vi "crio_FPGA_Antagonist_Force.vi"() -> ()   [LabVIEW 2019]
uses:
  <vilib>/rvi/Analysis/control/PID/Typedef/niFpgaPID_ManualControl.ctl
  <vilib>/rvi/Analysis/control/PID/Typedef/niFpgaPID_PIGains.ctl
  <vilib>/LabVIEW Targets/FPGA/cRIO/shared/nicrio_ModuleControls/nicrio_cRIO-9237_ExcitationVoltageRing.ctl
  <vilib>/LabVIEW Targets/FPGA/cRIO/shared/nicrio_ModuleControls/nicrio_cRIO-9237_DataRatesRing.ctl
  <vilib>/rvi/Analysis/control/PID/Typedef/niFpgaPID_OutputRange.ctl
  <vilib>/rvi/Emulation/niFpgaSctlEmulationGetInTimedLoop.vi
  <vilib>/rvi/Emulation/niFpgaProcessEmulError.vi
  <vilib>/rvi/eio/common/nirviEmuTemplateMethod_errors.vi
  <vilib>/rvi/eio/common/nirviEmuTemplatePropertySet_errors.vi
  <vilib>/rvi/Emulation/niFpgaGetClockAttributes.vi
  <vilib>/rvi/Emulation/niFpgaEmulationReportErrorSimple.vi
  <vilib>/rvi/Emulation/niFpgaCriticalErrorInLSC.vi
  <vilib>/rvi/Analysis/control/PID/SubVIs/niFpgaPID_PIWrapper.vi
  <vilib>/eio/EIOMethodNode/EIOMethodNode.xnode
  <vilib>/eio/EIOPropertyNode/EIOPropertyNode.xnode
  <vilib>/eio/EIONode/EIONode.xnode
  <vilib>/rvi/FXPMathLib/FxpInterpret/XNode/nifxpmath_Interpret.xnode
  <vilib>/rvi/FXPMathLib/FxpMul/XNode/nifxpmath_Multiplier.xnode
  <vilib>/rvi/FXPMathLib/FxpAdd/XNode/nifxpmath_Add.xnode
  <vilib>/rvi/eio/common/nirviEmuTemplatePropertyGet_errors.vi
  <vilib>/rvi/eio/common/nirviEmuTemplatePropertyGet_noerrors.vi
  <vilib>/rvi/eio/common/nirviEmuTemplatePropertySet_noerrors.vi
  <vilib>/rvi/FXPMathLib/sim/FxpSim.dll
panel:
  in  "sweep frequency (periods/tick)":fxp<+,32,0>=1.25030055642128e-06
  out "sine out":i16
  out "sin_fxp":fxp<+/-,16,1>
  out "cosine out":i16
  in  "Lock_loop_rate":u32 caption="Count(uSec)"
  in  "sin_gain":fxp<+,32,10>
  in  "sin_offset":fxp<+/-,32,10>=0.5
  out "VCA Force Setpoint":sgl
  out "scaled load cell reading":fxp<+/-,24,24>
  out "error out":errorcluster {"code" format="%.0x"}
  in  "Finite?":bool=TRUE
  in  "Samples per Channel":u32=1000
  out "Mod1/AI0":fxp<+/-,24,-4>
  in  "Loop Rate (uSec)":u32
  in  "Shunt Cal Enable":bool
  in  "Data Rate":T1=1 items=["50.000 kS/s (NI 9237)"=1, "25.000 kS/s (NI 9237)"=2, "16.667 kS/s (NI 9237)"=3, "12.500 kS/s (NI 9237)"=4, "10.000 kS/s (NI 9237)"=5, "8.333 kS/s (NI 9237)"=6, "7.143 kS/s (NI 9237)"=7, "6.250 kS/s (NI 9237)"=8, "5.556 kS/s (NI 9237)"=9, "5.000 kS/s (NI 9237)"=10, "4.545 kS/s (NI 9237)"=11, "4.167 kS/s (NI 9237)"=12, "3.846 kS/s (NI 9237)"=13, "3.571 kS/s (NI 9237)"=14, "3.333 kS/s (NI 9237)"=15, "3.125 kS/s (NI 9237)"=16, "2.941 kS/s (NI 9237)"=17, "2.778 kS/s (NI 9237)"=18, "2.632 kS/s (NI 9237)"=19, "2.500 kS/s (NI 9237)"=20, "2.381 kS/s (NI 9237)"=21, "2.273 kS/s (NI 9237)"=22, "2.174 kS/s (NI 9237)"=23, "2.083 kS/s (NI 9237)"=24, "2.000 kS/s (NI 9237)"=25, "1.923 kS/s (NI 9237)"=26, "1.852 kS/s (NI 9237)"=27, "1.786 kS/s (NI 9237)"=28, "1.724 kS/s (NI 9237)"=29, "1.667 kS/s (NI 9237)"=30, "1.613 kS/s (NI 9237)"=31]
  in  "Excitation Voltage":T2 items=["2.5 Volts", "3.3 Volts", "5.0 Volts", "10.0 Volts", "External Excitation"]
  in  "Half-Bridge Enable":bool
  in  "LAC Lock":bool
  in  "VCA Gains":T3 {"proportional gain" step=0.125}
  in  "LAC DC PWM Period (us)":i16=50
  in  "Debug: ConnectorA/DIO15":bool
  in  "Debug: ConnectorA/DIO14":bool
  in  "Encoder Debug":bool
  in  "Loop Timer DAQ":u32=1 caption="LAC Loop Time(uSec)"
  in  "Position Reset":bool
  out "LAC Position (Counts)":i32
  out "LAC B":bool
  out "LAC A":bool
  out "LAC B'":bool
  out "LAC A'":bool
  in  "LAC Velocity Interval (uSec)":u32=1000
  out "LAC Acceleration (Counts/Interval)":i32
  out "LAC Velocity (Counts/Interval)":i32
  out "LAC Controller PWM Output":sgl
  in  "LAC Manual Control":T4 {"manual input (0)" scale=-1.0..1.0}
  in  "LAC Setpoint":i32
  in  "LAC Gains":T3={"proportional gain"=0.01, "integral gain"=6e-09} {"proportional gain" step=0.125}
  in  "rail Initial Position":i16=1
  out "rail Platform Position":i16
  in  "Stepper Direction":bool
  in  "Stepper Enable":bool
  in  "Position Control: Desired Positoin":i16=100
  in  "Manual Operation":bool
  out "Controller Enable":bool
  out "Controller Direction":bool
  in  "mSec to initialize a small push away from limit switch":u32=1 caption="mSec when hit limit"
  in  "mSec when hit limit":u32=100 caption="rail mSec to pause when hit limit"
  in  "Rail soft limit":i16=10000
  out "Limit Switch":bool
  in  "Half Peirod (pulse 40MHz)":u32=10000 caption="rail Count(Tick) [Interval between step]"
  out "VCA ControllerPWM Output":sgl
  in  "VCA Manual Control":T4 {"manual input (0)" scale=-1.0..1.0}
  in  "DC PWM Period (microsec)":i16=50
  in  "stop":bool=TRUE
  # "Period Default 500(us) 2kHz"
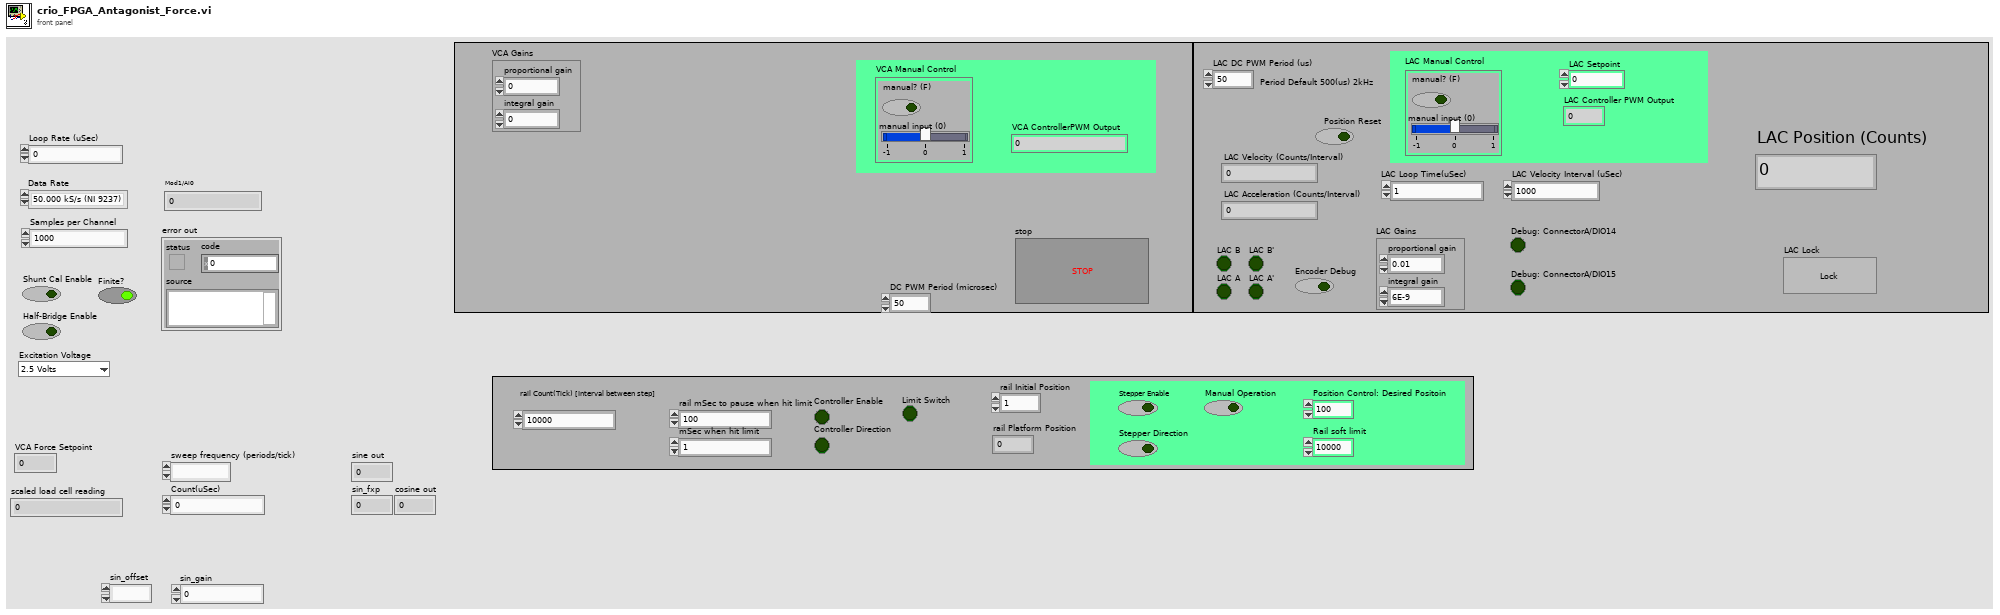
[diagram p1: front panel]
types:
  T1 = typedef "nicrio_cRIO-9237_DataRatesRing.ctl" = u8
  T2 = typedef "nicrio_cRIO-9237_ExcitationVoltageRing.ctl" = u8
  T3 = typedef "niFpgaPID_PIGains.ctl" = cluster{"proportional gain":sgl, "integral gain":sgl}
  T4 = typedef "niFpgaPID_ManualControl.ctl" = cluster{"manual? (F)":bool, "manual input (0)":sgl}
  T5 = typedef "niFpgaPID_OutputRange.ctl" = cluster{"output high (Inf)":sgl, "output low (-Inf)":sgl}
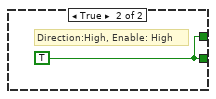
[diagram p6: hidden frame]
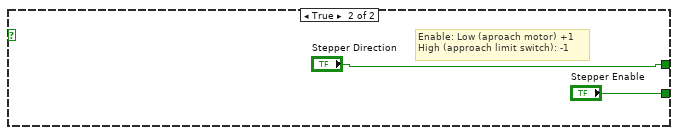
[diagram p7: hidden frame]
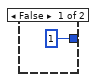
[diagram p9: hidden frame]
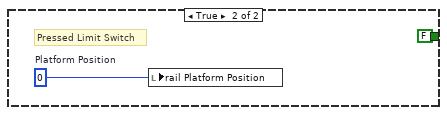
[diagram p11: hidden frame]
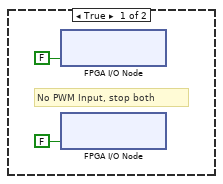
[diagram p13: hidden frame]
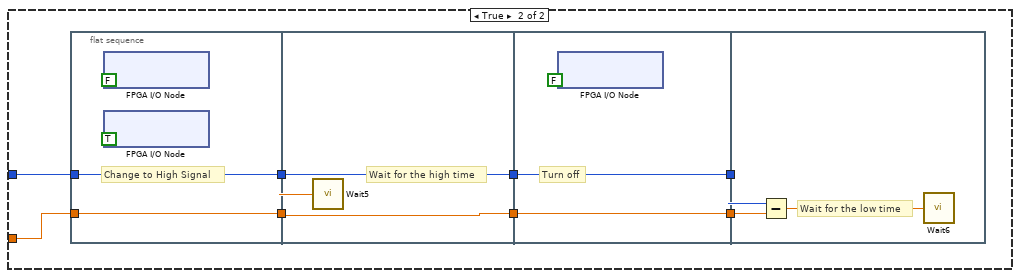
[diagram p14: hidden frame]
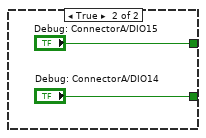
[diagram p17: hidden frame]
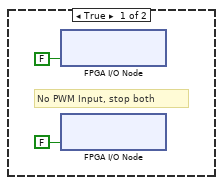
[diagram p18: hidden frame]
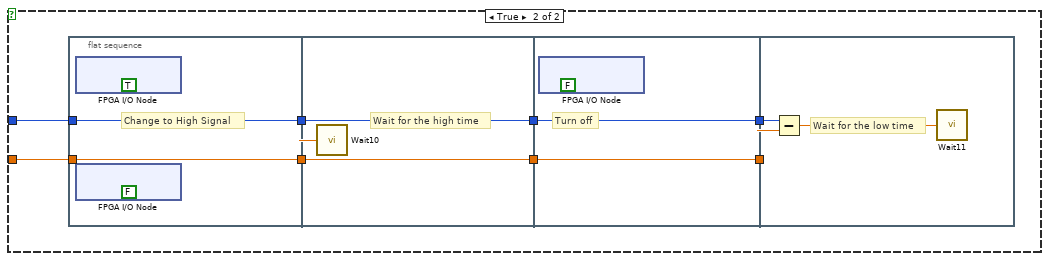
[diagram p19: hidden frame]
diagram:
  n1 = flat-sequence {
    tunnel: [w6] -> w2
    tunnel: [w5] -> w1
    tunnel: w2 -> [w30]
    tunnel: w1 -> [w29]
    frame #0 {
      n2 = disable-structure shown="Enabled" {
        disable-tunnel: [w17 _] -> w6
        disable-tunnel: ["Data Rate" _] -> w5
        frame Enabled {
          # "red to 2\ngreen to 3\nblack to 21\nwhite to 22"
          # "Start the Aquisition"
          # "For Quarter and Half Bridge strain gauges enable the half bridge \nto complete the full bridge."
          # "Set the modules data rate, acquisition rate, and excitation voltage."
          n3 = xnode "FPGA I/O Property Node"("error in"=errorcluster {"status"=FALSE, "code"=0, "source"=""}, "Data Rate"="Data Rate", "Excitation Voltage"="Excitation Voltage") -> ("error out"=w27:errorcluster)  [unwired: 1 in, 1 out]
          n4 = xnode "FPGA I/O Property Node"("error in"=w27, "Half-Bridge Enable"="Half-Bridge Enable") -> ("error out"=w23:errorcluster)  [unwired: 1 in, 1 out]
          n5 = xnode "FPGA I/O Property Node"("error in"=w27, "Half-Bridge Enable"="Half-Bridge Enable") -> ("error out"=w24:errorcluster)  [unwired: 1 in, 1 out]
          n6 = xnode "FPGA I/O Property Node"("error in"=w27, "Half-Bridge Enable"="Half-Bridge Enable") -> ("error out"=w25:errorcluster)  [unwired: 1 in, 1 out]
          n7 = xnode "FPGA I/O Property Node"("error in"=w27, "Half-Bridge Enable"="Half-Bridge Enable") -> ("error out"=w26:errorcluster)  [unwired: 1 in, 1 out]
          n8 = local write "Loop Rate (uSec)"(u32 100 ("Loop Rate (uSec)")) -> ()
          n9 = Merge Errors(w23, w24, w25, w26) -> (w28:errorcluster)
          n10 = xnode "FPGA I/O Node"("error in"=w28, "Mod6/Start"=TRUE ("Mod1/Stop")) -> ("error out"=w17:errorcluster)  [unwired: 1 in, 1 out]
        }
        frame Disabled {
        }
      }
      n11 = local write "scaled load cell reading"(0 ("LAC Position (Counts)")) -> ()
      n12 = local write "VCA Force Setpoint"(0 ("LAC Position (Counts)")) -> ()
      n13 = local write "stop"(FALSE ("stop")) -> ()
      n14 = xnode "FPGA I/O Method Node"("DIO 7:4"=enum8{"No Change", "Input", "Output"}."Input", "DIO 3:0"=enum8{"No Change", "Input", "Output"}."Output") -> ()  [unwired: 1 in, 1 out]
      n15 = local write "LAC Controller PWM Output"(u32 0 ("Servo wait time")) -> ()
      n16 = local write "LAC Position (Counts)"(0 ("LAC Position (Counts)")) -> ()
      n17 = local write "Encoder Debug"(FALSE ("LAC Lock")) -> ()
      n18 = local write "LAC Lock"(FALSE ("LAC Lock")) -> ()
      n19 = xnode "FPGA I/O Method Node"("Enable"=u8 0) -> ()  [unwired: 1 in, 1 out]
      "rail Platform Position" <- "rail Initial Position"
    }
    frame #1 {
      n20 = disable-structure shown="Enabled" {
        disable-tunnel: w30 -> [w32 _]
        disable-tunnel: w29 -> [w31 _]
        frame Enabled {
          n21 = while {
            stop <- w36 stop-if-true
            # "Shift by 20 bits"
            # "output"
            # "PWM"
            # "current offset"
            # "sine wave amplitude"
            # "Lock in"
            n22 = local read "Mod1/AI0"() -> (w35:fxp<+/-,24,-4>)
            n23 = call "Loop Timer2"("Count(uSec)"="Lock_loop_rate") -> ()  [unwired: 1 out]
            n24 = xnode "Reinterpret Number"("x"=w35) -> ("y"=→"scaled load cell reading":fxp<+/-,24,16>)
            n25 = call "Sine Wave Generator"("frequency (periods/tick)"="sweep frequency (periods/tick)") -> ("sine out"=w45:i16, "cosine out"=→"cosine out":i16)  [unwired: 13 in]
            "sine out" <- w45
            n26 = xnode "Reinterpret Number"("x"=w45) -> ("y"=w42:fxp<+/-,16,1>)
            "sin_fxp" <- w42
            n27 = xnode ("High Throughput Multiply")("x"=w42, "y"="sin_gain") -> ("x*y"=w40:fxp<+/-,48,11>)
            n28 = xnode ("High Throughput Add")("x"=w40, "y"="sin_offset") -> ("x+y"=w38:fxp<+/-,49,12>)
            n29 = To Single Precision Float(number=w38) -> (single precision float=→"VCA Force Setpoint":sgl)
            n30 = local read "stop"() -> (w36:bool)
          }
          n31 = flat-sequence {
            tunnel: [w49] -> w33
            tunnel: w32 -> [w48]
            tunnel: w31 -> [w47]
            tunnel: w33 -> [w118]
            frame #0 {
              # "Stop on any error or if the stop Boolean is true"
              n32 = while {
                tunnel: w48 -> [w60]
                tunnel: [w57] -> w49
                tunnel: w47 -> [w55]
                stop <- w58 stop-if-true
                n33 = flat-sequence {
                  tunnel: [w63] -> w56
                  tunnel: [w62] -> w53
                  tunnel: ["Shunt Cal Enable"] -> w52
                  tunnel: w55 -> [w62]
                  tunnel: w60 -> [w64]
                  tunnel: [w81] -> w59
                  tunnel: w56 -> [w82]
                  tunnel: [w80] -> w54
                  tunnel: w53 -> [w80]
                  tunnel: w52 -> [w79]
                  tunnel: [w79] -> w51
                  tunnel: [w101] -> w57
                  tunnel: w59 -> [w102]
                  tunnel: w54 -> [w99]
                  tunnel: w51 -> [w100]
                  frame #0 {
                    n34 = case shown="True" "Shunt Cal Enable" {
                      tunnel: w64 -> [w65 w75]
                      tunnel: [w65 w73] -> w63
                      tunnel: w62 -> [_ w70]
                      frame False {
                      }
                      frame True {
                        w68 = TRUE ("Shunt Cal Enable")
                        # "If Shunt Cal Enable is true stop the acquisition, switch on the shunt resistors, set the data rate and begin the acquisition."
                        n35 = xnode "FPGA I/O Node"("error in"=w75, "Mod6/Stop"=TRUE ("Mod1/Stop")) -> ("error out"=w74:errorcluster)  [unwired: 1 in, 1 out]
                        n36 = xnode "FPGA I/O Property Node"("error in"=w74, "Shunt Cal Enable"=w68) -> ("error out"=w78:errorcluster)  [unwired: 1 in, 1 out]
                        n37 = xnode "FPGA I/O Property Node"("error in"=w74, "Shunt Cal Enable"=w68) -> ("error out"=w66:errorcluster)  [unwired: 1 in, 1 out]
                        n38 = xnode "FPGA I/O Property Node"("error in"=w74, "Shunt Cal Enable"=w68) -> ("error out"=w77:errorcluster)  [unwired: 1 in, 1 out]
                        n39 = xnode "FPGA I/O Property Node"("error in"=w74, "Shunt Cal Enable"=w68) -> ("error out"=w76:errorcluster)  [unwired: 1 in, 1 out]
                        n40 = Merge Errors(w78, w66, w77, w76) -> (w71:errorcluster)
                        n41 = xnode "FPGA I/O Property Node"("error in"=w71, "Data Rate"=w70) -> ("error out"=w72:errorcluster)  [unwired: 1 in, 1 out]
                        n42 = xnode "FPGA I/O Node"("error in"=w72, "Mod6/Start"=TRUE ("Mod1/Start")) -> ("error out"=w73:errorcluster)  [unwired: 1 in, 1 out]
                      }
                    }
                  }
                  frame #1 {
                    n43 = while {
                      tunnel: w82 -> [w84]
                      tunnel: [w88] -> w81
                      i -> [w92]
                      stop <- w85 stop-if-true
                      # "When the Finite Boolean is true the code will acquire a discrete set of values in order to perform the offset null and/or shunt calibration otherwise the loop continuously acquires data."
                      n44 = Decrement(x="Samples per Channel") -> (x-1=w94:u32)
                      n45 = call "Loop Timer3"("Count(uSec)"="Loop Rate (uSec)") -> ()  [unwired: 1 out]
                      n46 = To Unsigned Long Integer(number=w92) -> (unsigned 32bit integer=w93:u32)
                      n47 = Equal?(x=w94, y=w93) -> (x = y?=w89:bool)
                      n48 = xnode "FPGA I/O Node"("error in"=w84) -> ("error out"=w88:errorcluster, "Mod6/AI0"=w98:fxp<+/-,24,-4>, "Mod6/AI1"=w97:fxp<+/-,24,-4>, "Mod6/AI2"=w95:fxp<+/-,24,-4>, "Mod6/AI3"=w96:fxp<+/-,24,-4>)  [unwired: 4 in, 4 out]
                      "Mod1/AI0" <- w98
                      n49 = And(x="Finite?", y=w89) -> (x .and. y?=w87:bool)
                      n50 = Build Array(w98, w97, w95, w96) -> ()  [unwired: 1 out]
                      n51 = local read "stop"() -> (w86:bool)
                      n52 = Compound Arithmetic op=OR(w88, w87, w86) -> (w85:bool)
                    }
                  }
                  frame #2 {
                    n53 = case shown="True" w100 {
                      tunnel: w102 -> [w103 w112]
                      tunnel: [w103 w110] -> w101
                      tunnel: w99 -> [_ w107]
                      frame False {
                      }
                      frame True {
                        w106 = FALSE ("Shunt Cal Enable")
                        # "If shunt calibration is set to true, data has been collected to perform the calibration. Next the acquisition is stopped, and then we switch off the shunt resistors, set the data rate, and start the acquisition."
                        n54 = xnode "FPGA I/O Node"("error in"=w112, "Mod6/Stop"=TRUE ("Mod1/Stop")) -> ("error out"=w111:errorcluster)  [unwired: 1 in, 1 out]
                        n55 = xnode "FPGA I/O Property Node"("error in"=w111, "Shunt Cal Enable"=w106) -> ("error out"=w116:errorcluster)  [unwired: 1 in, 1 out]
                        n56 = xnode "FPGA I/O Property Node"("error in"=w111, "Shunt Cal Enable"=w106) -> ("error out"=w115:errorcluster)  [unwired: 1 in, 1 out]
                        n57 = xnode "FPGA I/O Property Node"("error in"=w111, "Shunt Cal Enable"=w106) -> ("error out"=w114:errorcluster)  [unwired: 1 in, 1 out]
                        n58 = xnode "FPGA I/O Property Node"("error in"=w111, "Shunt Cal Enable"=w106) -> ("error out"=w113:errorcluster)  [unwired: 1 in, 1 out]
                        n59 = Merge Errors(w116, w115, w114, w113) -> (w108:errorcluster)
                        n60 = xnode "FPGA I/O Property Node"("error in"=w108, "Data Rate"=w107) -> ("error out"=w109:errorcluster)  [unwired: 1 in, 1 out]
                        n61 = xnode "FPGA I/O Node"("error in"=w109, "Mod6/Start"=TRUE ("Mod1/Start")) -> ("error out"=w110:errorcluster)  [unwired: 1 in, 1 out]
                      }
                    }
                  }
                }
                n62 = local read "stop"() -> (w50:bool)
                n63 = Or(x=w57, y=w50) -> (x .or. y?=w58:bool)
              }
            }
            frame #1 {
              # "Stop the acquisition and display any errors that occurred."
              n64 = xnode "FPGA I/O Node"("error in"=w118, "Mod6/Stop"=TRUE ("Mod1/Stop")) -> ("error out"=→"error out":errorcluster)  [unwired: 1 in, 1 out]
            }
          }
        }
        frame Disabled {
        }
      }
      n65 = disable-structure "LAC Position Control" shown="Enabled" {
        frame Enabled {
          n66 = while "Input Loop" {
            shift-right: [w254] -> _
            shift-left: _ -> [w257]
            shift-right: [w253] -> _
            shift-left: _ -> [w256]
            shift-right: [w249] -> _
            shift-left: _ -> [w255]
            shift-right: [w242] -> _
            shift-left: _ -> [w252]
            shift-right: [w243] -> _
            shift-left: _ -> [w251]
            shift-right: [w250] -> _
            shift-left: _ -> [w248]
            shift-right: [w247] -> _
            shift-left: _ -> [w246]
            shift-right: [w245] -> _
            shift-left: _ -> [w244]
            stop <- w241 stop-if-true
            # "B'"
            # ">>ChB>>"
            # ">>ChA>>"
            # "A'"
            # "A  -> Current Quadrature Encoder Channel A value\nA' -> Last value of Quadrature Encoder Channel A\nB  -> Current Quadrature Encoder Channel B value\nB' -> Last value of Quadrature Encoder Channel B"
            # "B'"
            # "B"
            # "A"
            n67 = case "Debug Input" shown="False" "Encoder Debug" {
              tunnel: [w275 "Debug: ConnectorA/DIO15"] -> w253
              tunnel: [w274 "Debug: ConnectorA/DIO14"] -> w254
              frame False {
                n68 = xnode "FPGA I/O Node"() -> ("Mod2/DIO2"=w275:bool, "Mod2/DIO3"=w274:bool)  [unwired: 2 in, 2 out]
              }
              frame True {
              }
            }
            "LAC B" <- w254
            "LAC A" <- w253
            n69 = call "Loop Timer"("Count(uSec)"="Loop Timer DAQ") -> ()  [unwired: 1 out]
            n70 = call "subvi_encoder_update.vi"("Position Reset"="Position Reset", "Tick'"=w255, "A"=w253, "B'"=w257, "A'"=w256, "B"=w254) -> ("Tick"=w249:i32)  [unwired: 5 in]
            "LAC Position (Counts)" <- w249
            n71 = disable-structure shown="Enabled" {
              disable-tunnel: w252 -> [w272 _]
              disable-tunnel: w251 -> [w271 _]
              disable-tunnel: [w270 _] -> w250
              disable-tunnel: w249 -> [w269 _]
              disable-tunnel: w248 -> [w268 _]
              disable-tunnel: [w267 _] -> w247
              disable-tunnel: w246 -> [w266 _]
              disable-tunnel: [w265 _] -> w245
              disable-tunnel: w244 -> [w264 _]
              disable-tunnel: [w262 _] -> w243
              disable-tunnel: [w261 _] -> w242
              frame Enabled {
                n72 = call "Time Count"() -> ("Tick Count(uSec)"=w263:u32)
                n73 = call "subvi_encoder_tick_to_pos.vi"("Velocity Interval (uSec)"="LAC Velocity Interval (uSec)", "Raw Tick"=w269, "Waited?'"=w266, "Tick Count(uSec)'"=w264, "p'"=w268, "Time Count"=w263, "a'"=w271, "v'"=w272) -> ("Waited?"=w267:bool, "Tick Count(uSec)"=w265:u32, "p"=w270:i32, "a"=w262:i32, "v"=w261:i32)  [unwired: 3 in]
                "LAC Acceleration (Counts/Interval)" <- w262
                "LAC Velocity (Counts/Interval)" <- w261
              }
              frame Disabled {
              }
            }
            n74 = local read "stop"() -> (w241:bool)
            "LAC B'" <- w257
            "LAC A'" <- w256
          }
          n75 = while {
            stop <- w240 stop-if-true
            n76 = local read "LAC Position (Counts)"() -> (w239:i32)
            n77 = call-poly <vilib>:"niFpgaPID_Wrapper.vi"("setpoint"="LAC Setpoint", "process variable"=w239, "manual control"="LAC Manual Control", "gains"="LAC Gains", "output range"=T5 {"output high (Inf)"=1.0, "output low (-Inf)"=-1.0}) -> ("output"=→"LAC Controller PWM Output":sgl)  [unwired: 8 in, 2 out]
            n78 = local read "stop"() -> (w240:bool)
          }
          n79 = while "PWM Output Loop" {
            stop <- w278 stop-if-true
            # "PWM input range:\n[-1,1]"
            # "DRV8256 Specs:\n\n0 0: Brake Low\n1 1: Brake High\nPWM 0\n0 PWM"
            # "controller output"
            n80 = local read "LAC Controller PWM Output"() -> (w279:sgl)
            n81 = Multiply(x="LAC DC PWM Period (us)", y=w279) -> (x*y=w281:sgl)
            n82 = Greater?(x=w279, y=i16 0) -> (0:w282:bool)
            n83 = case shown="False" w282 {
              tunnel: w281 -> [w286 w317]
              tunnel: "LAC DC PWM Period (us)" -> [w284 w316]
              frame False {
                n84 = Equal To 0?(x=w286) -> (x = 0?=w285:bool)
                n85 = case shown="False" w285 {
                  tunnel: w286 -> [_ w296]
                  tunnel: w284 -> [_ w289]
                  frame True {
                    # "No PWM Input, stop both"
                    n86 = xnode "FPGA I/O Node"("Mod1/DIO2"=FALSE) -> ()  [unwired: 1 in, 1 out]
                    n87 = xnode "FPGA I/O Node"("Mod1/DIO3"=FALSE) -> ()  [unwired: 1 in, 1 out]
                  }
                  frame False {
                    # "Negative duty cycle (change direction by outputting to other PIN)"
                    n88 = flat-sequence {
                      tunnel: w296 -> [w299]
                      tunnel: [w298] -> w295
                      tunnel: [w297] -> w290
                      tunnel: w289 -> [w297]
                      tunnel: w295 -> [w303]
                      tunnel: [w303] -> w294
                      tunnel: [w302] -> w291
                      tunnel: w290 -> [w302]
                      tunnel: w294 -> [w305]
                      tunnel: [w305] -> w293
                      tunnel: [w304] -> w292
                      tunnel: w291 -> [w304]
                      tunnel: w293 -> [w309]
                      tunnel: w292 -> [w308]
                      frame #0 {
                        # "Change to High Signal"
                        n89 = xnode "FPGA I/O Node"("Mod1/DIO3"=TRUE) -> ()  [unwired: 1 in, 1 out]
                        n90 = xnode "FPGA I/O Node"("Mod1/DIO2"=FALSE) -> ()  [unwired: 1 in, 1 out]
                        n91 = Negate(x=w299) -> (-x=w298:sgl)
                      }
                      frame #1 {
                        # "Wait for the High Time"
                        n92 = call "Wait"("Count(uSec)"=w303) -> ()  [unwired: 1 out]
                      }
                      frame #2 {
                        # "Change to Low Signal"
                        n93 = xnode "FPGA I/O Node"("Mod1/DIO2"=FALSE) -> ()  [unwired: 1 in, 1 out]
                      }
                      frame #3 {
                        # "Wait for the low time"
                        n94 = Subtract(x=w308, y=w309) -> (x-y=w307:sgl)
                        n95 = call "Wait2"("Count(uSec)"=w307) -> ()  [unwired: 1 out]
                      }
                    }
                  }
                }
              }
              frame True {
                n96 = flat-sequence {
                  tunnel: w317 -> [w318]
                  tunnel: w316 -> [w319]
                  tunnel: [w319] -> w313
                  tunnel: [w318] -> w312
                  tunnel: [w323] -> w314
                  tunnel: w313 -> [w323]
                  tunnel: w312 -> [w322]
                  tunnel: [w322] -> w311
                  tunnel: [w325] -> w315
                  tunnel: w314 -> [w325]
                  tunnel: w311 -> [w324]
                  tunnel: [w324] -> w310
                  tunnel: w315 -> [w329]
                  tunnel: w310 -> [w327]
                  frame #0 {
                    # "Change to High Signal"
                    n97 = xnode "FPGA I/O Node"("Mod1/DIO2"=TRUE) -> ()  [unwired: 1 in, 1 out]
                    n98 = xnode "FPGA I/O Node"("Mod1/DIO3"=FALSE ("ConnectorB/DIO9")) -> ()  [unwired: 1 in, 1 out]
                  }
                  frame #1 {
                    # "Wait for the high time"
                    n99 = call "Wait10"("Count(uSec)"=w322) -> ()  [unwired: 1 out]
                  }
                  frame #2 {
                    # "Turn off"
                    n100 = xnode "FPGA I/O Node"("Mod1/DIO2"=FALSE) -> ()  [unwired: 1 in, 1 out]
                  }
                  frame #3 {
                    # "Wait for the low time"
                    n101 = Subtract(x=w329, y=w327) -> (x-y=w328:sgl)
                    n102 = call "Wait11"("Count(uSec)"=w328) -> ()  [unwired: 1 out]
                  }
                }
              }
            }
            n103 = local read "stop"() -> (w278:bool)
          }
          n104 = while {
            stop <- w233 stop-if-true
            # "Lock the LAC controller with relay.\nRelay pin HIGH means connects to ground, meaning LAC powered OFF."
            n105 = xnode "FPGA I/O Node"("Mod8/DIO6"="LAC Lock") -> ()  [unwired: 1 in, 1 out]
            n106 = local read "stop"() -> (w233:bool)
          }
        }
        frame Disabled {
        }
      }
      n107 = disable-structure "VCA Control" shown="Enabled" {
        frame Enabled {
          n108 = while {
            stop <- w179 stop-if-true
            n109 = local read "scaled load cell reading"() -> (w174:fxp<+/-,24,24>)
            n110 = local read "VCA Force Setpoint"() -> (w173:sgl)
            n111 = call-poly <vilib>:"niFpgaPID_Wrapper.vi"("setpoint"=w173, "process variable"=w174, "manual control"="VCA Manual Control", "gains"="VCA Gains", "output range"=T5 {"output high (Inf)"=1.0, "output low (-Inf)"=-1.0}) -> ("output"=→"VCA ControllerPWM Output":sgl)  [unwired: 8 in, 2 out]
            n112 = local read "stop"() -> (w179:bool)
          }
          n113 = while "PWM Output Loop" {
            stop <- w180 stop-if-true
            # "PWM input range:\n[-1,1]"
            # "DRV8256 Specs:\n\n0 0: Brake Low\n1 1: Brake High\nPWM 0\n0 PWM"
            # "controller output"
            n114 = local read "VCA ControllerPWM Output"() -> (w181:sgl)
            n115 = Greater?(x=w181, y=i16 0) -> (0:w184:bool)
            n116 = Multiply(x="DC PWM Period (microsec)", y=w181) -> (x*y=w183:sgl)
            n117 = case shown="False" w184 {
              tunnel: w183 -> [w188 w219]
              tunnel: "DC PWM Period (microsec)" -> [w186 w218]
              frame False {
                n118 = Equal To 0?(x=w188) -> (x = 0?=w187:bool)
                n119 = case shown="False" w187 {
                  tunnel: w188 -> [_ w198]
                  tunnel: w186 -> [_ w191]
                  frame True {
                    # "No PWM Input, stop both"
                    n120 = xnode "FPGA I/O Node"("Mod1/DIO1"=FALSE) -> ()  [unwired: 1 in, 1 out]
                    n121 = xnode "FPGA I/O Node"("Mod1/DIO0"=FALSE) -> ()  [unwired: 1 in, 1 out]
                  }
                  frame False {
                    # "Negative duty cycle (change direction by outputting to other PIN)"
                    n122 = flat-sequence {
                      tunnel: w198 -> [w201]
                      tunnel: [w200] -> w197
                      tunnel: [w199] -> w192
                      tunnel: w191 -> [w199]
                      tunnel: w197 -> [w205]
                      tunnel: [w205] -> w196
                      tunnel: [w204] -> w193
                      tunnel: w192 -> [w204]
                      tunnel: w196 -> [w207]
                      tunnel: [w207] -> w195
                      tunnel: [w206] -> w194
                      tunnel: w193 -> [w206]
                      tunnel: w195 -> [w211]
                      tunnel: w194 -> [w210]
                      frame #0 {
                        # "Change to High Signal"
                        n123 = Negate(x=w201) -> (-x=w200:sgl)
                        n124 = xnode "FPGA I/O Node"("Mod1/DIO1"=TRUE) -> ()  [unwired: 1 in, 1 out]
                        n125 = xnode "FPGA I/O Node"("Mod1/DIO0"=FALSE) -> ()  [unwired: 1 in, 1 out]
                      }
                      frame #1 {
                        # "Wait for the High Time"
                        n126 = call "Wait3"("Count(uSec)"=w205) -> ()  [unwired: 1 out]
                      }
                      frame #2 {
                        # "Change to Low Signal"
                        n127 = xnode "FPGA I/O Node"("Mod1/DIO1"=FALSE) -> ()  [unwired: 1 in, 1 out]
                      }
                      frame #3 {
                        # "Wait for the low time"
                        n128 = Subtract(x=w210, y=w211) -> (x-y=w209:sgl)
                        n129 = call "Wait4"("Count(uSec)"=w209) -> ()  [unwired: 1 out]
                      }
                    }
                  }
                }
              }
              frame True {
                n130 = flat-sequence {
                  tunnel: w219 -> [w220]
                  tunnel: w218 -> [w221]
                  tunnel: [w221] -> w215
                  tunnel: [w220] -> w214
                  tunnel: [w225] -> w216
                  tunnel: w215 -> [w225]
                  tunnel: w214 -> [w224]
                  tunnel: [w224] -> w213
                  tunnel: [w227] -> w217
                  tunnel: w216 -> [w227]
                  tunnel: w213 -> [w226]
                  tunnel: [w226] -> w212
                  tunnel: w217 -> [w231]
                  tunnel: w212 -> [w229]
                  frame #0 {
                    # "Change to High Signal"
                    n131 = xnode "FPGA I/O Node"("Mod1/DIO1"=FALSE ("ConnectorB/DIO9")) -> ()  [unwired: 1 in, 1 out]
                    n132 = xnode "FPGA I/O Node"("Mod1/DIO0"=TRUE) -> ()  [unwired: 1 in, 1 out]
                  }
                  frame #1 {
                    # "Wait for the high time"
                    n133 = call "Wait5"("Count(uSec)"=w224) -> ()  [unwired: 1 out]
                  }
                  frame #2 {
                    # "Turn off"
                    n134 = xnode "FPGA I/O Node"("Mod1/DIO0"=FALSE) -> ()  [unwired: 1 in, 1 out]
                  }
                  frame #3 {
                    # "Wait for the low time"
                    n135 = Subtract(x=w231, y=w229) -> (x-y=w230:sgl)
                    n136 = call "Wait6"("Count(uSec)"=w230) -> ()  [unwired: 1 out]
                  }
                }
              }
            }
            n137 = local read "stop"() -> (w180:bool)
          }
        }
        frame Disabled {
        }
      }
      n138 = while {
        stop <- "stop" stop-if-true
      }
      n139 = disable-structure "Rail" shown="Enabled" {
        frame Enabled {
          n140 = while "Limit Swtich Input" {
            stop <- w171 stop-if-true
            (unwired) TRUE ("Mod8/DIO2")
            n141 = xnode "FPGA I/O Node"() -> ("Mod8/DIO2"=w172:bool)  [unwired: 1 in, 1 out]
            "Limit Switch" <- w172
            n142 = local write "Limit Switch"(w172) -> ()
            n143 = local read "stop"() -> (w171:bool)
          }
          n144 = while "Drive" {
            stop <- w139 stop-if-true
            # "Direction: Low (aproach motor) +1\nHigh (approach limit switch): -1"
            n145 = local read "Controller Direction"() -> (w140:bool)
            n146 = local read "rail Platform Position"() -> (w142:i16)
            n147 = local read "Controller Enable"() -> (w141:bool)
            n148 = xnode "FPGA I/O Node"("Mod8/DIO4"=w140) -> ()  [unwired: 1 in, 1 out]
            n149 = case shown="True" w141 {
              tunnel: w140 -> [_ w147]
              tunnel: w142 -> [_ w144]
              frame False {
              }
              frame True {
                n150 = case shown="True" w147 {
                  tunnel: [i16 1 i16 -1] -> w146
                  frame False {
                  }
                  frame True {
                    # "Stepper Moving"
                  }
                }
                n151 = feedback #1(FALSE ("Connector0/DIO0")) -> (w148:bool)
                n152 = xnode "FPGA I/O Node"("Mod8/DIO3"=w148) -> ()  [unwired: 1 in, 1 out]
                n153 = Not(x=w148) -> (.not. x?=w149:bool)
                n154 = feedback-in #1(w149) -> ()
                n155 = Add(x=w144, y=w146) -> (x+y=w145:i16)
                n156 = local write "rail Platform Position"(w145) -> ()
              }
            }
            n157 = call "Wait7"("Count(Ticks)"="Half Peirod (pulse 40MHz)") -> ()  [unwired: 1 out]
            n158 = local read "stop"() -> (w139:bool)
          }
          n159 = while "Controller Loop" {
            stop <- w124 stop-if-true
            n160 = case shown="False" "Manual Operation" {
              tunnel: [w128 "Stepper Enable"] -> w122
              tunnel: [w127 "Stepper Direction"] -> w121
              frame False {
                n161 = local read "rail Platform Position"() -> (w125:i16)
                n162 = Greater?(x=w125, y="Position Control: Desired Positoin") -> (0:w129:bool)
                n163 = case shown="False" w129 {
                  tunnel: [w132 w136] -> w128
                  tunnel: [w130 w136] -> w127
                  tunnel: "Position Control: Desired Positoin" -> [w135 _]
                  tunnel: w125 -> [w134 _]
                  frame False {
                    w130 = FALSE
                    n164 = Equal?(x=w134, y=w135) -> (x = y?=w133:bool)
                    n165 = Select(t=w130, s=w133, f=TRUE) -> (s? t:f=w132:bool)
                  }
                  frame True {
                    w136 = TRUE
                    # "Direction:High, Enable: High"
                  }
                }
              }
              frame True {
                # "Enable: Low (aproach motor) +1\nHigh (approach limit switch): -1"
              }
            }
            "Controller Enable" <- w122
            "Controller Direction" <- w121
            n166 = local read "stop"() -> (w124:bool)
          }
          n167 = while "Handling Limits" {
            stop <- w159 stop-if-true
            # "False means touched"
            n168 = local read "rail Platform Position"() -> (w158:i16)
            n169 = local read "Limit Switch"() -> (w154:bool)
            n170 = Greater?(x=w158, y="Rail soft limit") -> (0:w156:bool)
            n171 = Not(x=w154) -> (.not. x?=w153:bool)
            n172 = Or(x=w153, y=w156) -> (x .or. y?=w155:bool)
            n173 = case shown="True" w155 {
              tunnel: w153 -> [_ w160]
              frame False {
                # "Do nothing"
              }
              frame True {
                n174 = flat-sequence {
                  tunnel: w160 -> [w161]
                  frame #0 {
                    # "Switch direction and shut off to prevent from going, and wait for some ms before moving."
                    n175 = case shown="False" w161 {
                      tunnel: [TRUE ("Stepper Direction") FALSE ("Stepper Direction")] -> w162
                      frame False {
                        # "Exceeds soft limit, change direction to approach switch"
                      }
                      frame True {
                        w167 = i16 0  # Platform Position
                        # "Pressed Limit Switch"
                        n176 = local write "rail Platform Position"(w167) -> ()
                      }
                    }
                    n177 = local write "Controller Enable"(FALSE ("Stepper Direction")) -> ()
                    n178 = call "Wait8"("Count(mSec)"="mSec when hit limit") -> ()  [unwired: 1 out]
                    n179 = local write "Controller Direction"(w162) -> ()
                  }
                  frame #1 {
                    # "Initialize a small push away from limit switch"
                    n180 = local write "Controller Enable"(TRUE ("Stepper Enable")) -> ()
                    n181 = call "Wait9"("Count(mSec)"="mSec to initialize a small push away from limit switch") -> ()  [unwired: 1 out]
                  }
                  frame #2 {
                    # "Stationary."
                    n182 = local write "Controller Enable"(FALSE ("Stepper Enable")) -> ()
                  }
                }
              }
            }
            n183 = local read "stop"() -> (w159:bool)
          }
        }
        frame Disabled {
        }
      }
    }
    frame #2 {
    }
  }
